vi "getDB Wafer Info.vi"(8 "error in (no error)":errorcluster, 10 "DSN":string="DSN=behemoth-new", 11 "Wafer Name":string="411-7556-5-A") -> (0 "error out":errorcluster, 3 "WaferInfo":T1)   [LabVIEW 2012]
panel:
  out "sql string":string
  in  "WaferInfo 2":T1
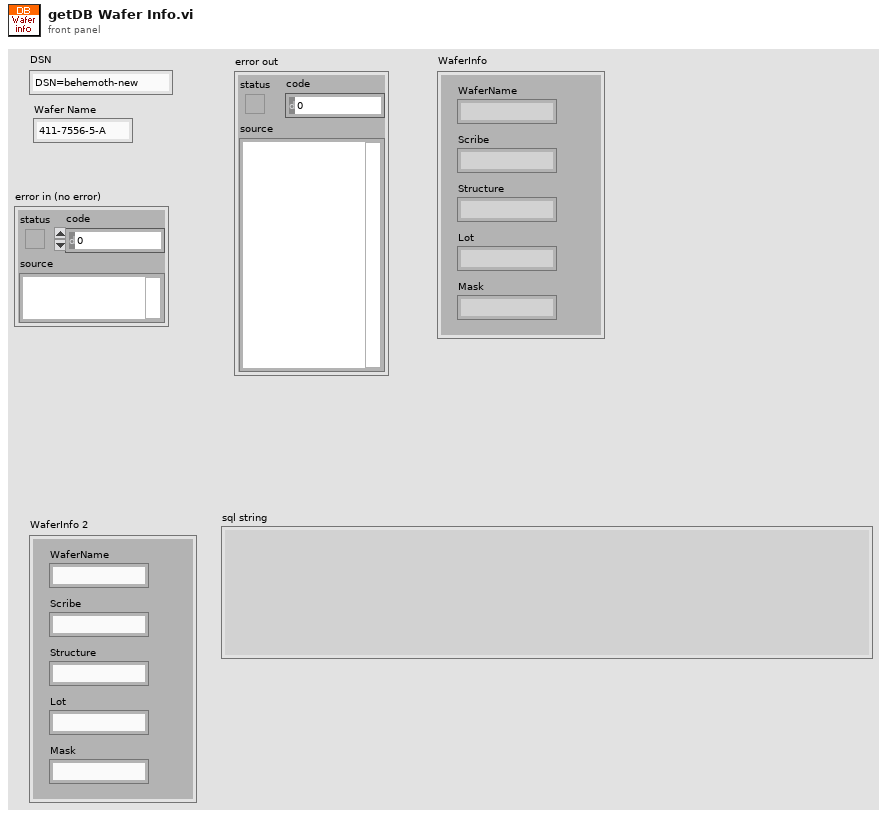
[diagram p1: front panel]
types:
  T1 = cluster{"WaferName":string, "Scribe":string, "Structure":string, "Lot":string, "Mask":string}
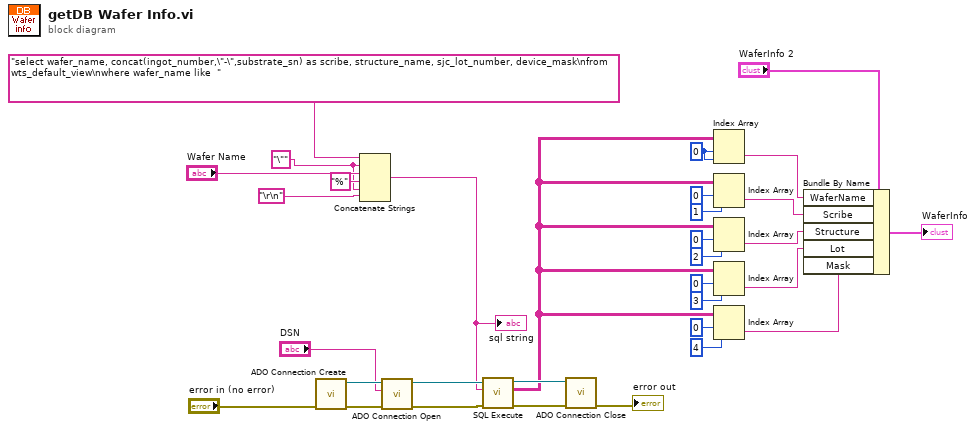
[diagram p0: block diagram]
diagram:
  w18 = 0 ("index (row)")
  w21 = "\""
  n1 = call "ADO Connection Create.vi"("error in (no error)"="error in (no error)") -> ("error out"=w30:errorcluster, "ADODB._Connection Out"=w31:refnum<k7>)  [unwired: 9 in]
  n2 = Concatenate Strings("select wafer_name, concat(ingot_number,\"-\",substrate_sn) as scribe, structure_name, sjc_lot_number, device_mask\nfrom wts_default_view\nwhere wafer_name like  ", w21, "Wafer Name", "%" ("string"), w21, "\r\n") -> (w19:string)
  "sql string" <- w19
  n3 = call "ADO Connection Open.vi"("error in (no error)"=w30, "ConnectionString"="DSN", "ADODB._Connection In"=w31) -> ("error out"=w28:errorcluster, "ADODB._Connection Out"=w29:refnum<k7>)  [unwired: 7 in]
  n4 = call "SQL Execute.vi"("error in (no error)"=w28, "Command Text"=w19, "ADODB._Connection In"=w29) -> ("error out"=w26:errorcluster, "Data"=w11:string[][], "ADODB._Connection Out"=w27:refnum<k7>)  [unwired: 5 in, 1 out]
  n5 = call "ADO Connection Close.vi"("error in (no error)"=w26, "ADODB._Connection In"=w27) -> ("error out"=→"error out":errorcluster)  [unwired: 8 in, 1 out]
  n6 = Index Array(array=w11, index (row)=w18, index (col)=w18) -> (element=w7:string)
  n7 = Index Array(array=w11, index (row)=0, index (col)=1 ("disabled index (col)")) -> (element=w6:string)
  n8 = Index Array(array=w11, index (row)=0, index (col)=2 ("disabled index (col)")) -> (element=w5:string)
  n9 = Index Array(array=w11, index (row)=0, index (col)=3 ("disabled index (col)")) -> (element=w4:string)
  n10 = Index Array(array=w11, index (row)=0, index (col)=4 ("disabled index (col)")) -> (element=w3:string)
  n11 = Bundle By Name(cluster="WaferInfo 2", "WaferName"=w7, "Scribe"=w6, "Structure"=w5, "Lot"=w4, "Mask"=w3) -> (→"WaferInfo":T1)
